vi "FTSMain.vi"() -> ()   [LabVIEW 2020]
uses:
  Popup/Transparent Button.ctl
  Main Menu Selector.ctl
  <instrlib>/PalmSens SDK for LabVIEW 5.10/PalmSens/LiveCurveResult.ctl
  support/PCT FGV CMD.ctl
  support/Message Queue/Message Cluster.ctl
  support/Message Queue/Enqueue Message (Single).vi
  <vilib>/ErrorRing/Error Ring.xnode
  <instrlib>/PalmSens SDK for LabVIEW 5.10/PalmSens/PalmSens.lvclass
  support/Message Queue/Message Queue.lvlib
  Popup/Popup Dialog.lvlib
panel:
  out "Pump Status":bool caption="Pressure"
  out "MFC Status":bool caption="Pressure"
  out "Hiden Status":bool caption="Pressure"
  in  "PS Live Curve Result":T1={"X Label"="Time", "Y Label"="Current", "Name"="Chronoamperometry: CA i vs t", "Index"=0, "Curve Values"={"Values"=array[20001 elements], "Index"=0}}
  in  "Start Motor":bool=TRUE caption="STOP Motor"
  out "Palm Sense Measuring":bool
  out "PS Status":bool caption="Pressure"
  out "User Details":string="Resticted " caption="щн дбегч"
  in  "Multicolumn Listbox":i32(listbox)=1
  out "Motor Status":bool caption="DB"
  in  "Main Menu":T2
  out "String 9":string="V 2.0.2"
  in  "String 7":string="S/N 123456"
  in  "String 6":string="P/N 123456"
  in  "String 5":string="Test Stand"
  out "Time Display":string="12:15:10"
  out "Date Display":string="12.11.2021"
  out "info":string caption="щн дбегч"
  out "Transparent":T3
  in  "Act Log 2":string
  in  "Spare":bool=TRUE caption="StartHeating"
  in  "Test 2":bool=TRUE caption="RUN_Test"
  out "Waveform Graph":dbl[](graph)
  in  "Report":bool
  in  "Timer Run":bool
  in  "CHANNEL 2":bool[](array[boolean])
  out "Display Tab":enum32{"Test", "History"}(tab)
  in  "Start Scan":bool caption="Start Process"
  in  "PS Save Measurements":bool=TRUE caption="RUN_Test"
  out "PS Data":cluster{"X":dbl[], "Y":dbl[]}[](graph)
  out "PS XY Graph":cluster{"X":dbl, "Y":dbl}[](graph)
  out "Waveform Chart 2":dbl[](graph)
  out "SP List Ind":i32(listbox)
  in  "Manual Tab":enum32{"Tango", "PalmSens", "MFC", "Pump"}(tab)
  in  "XYZ Velocity":dbl
  out "Actual Position":cluster{"dX":dbl, "dY":dbl, "dZ":dbl, "dA":dbl}={"dX"=150.0, "dY"=150.0, "dZ"=150.0, "dA"=0.0} caption="Actual Pos\n[mm]"
  in  "Position Mode":string(combo)="Absolute"
  in  "Motor Home":bool=TRUE caption="RUN_Test"
  in  "Set Position":cluster{"dX":dbl, "dY":dbl, "dZ":dbl, "dA":dbl} caption="Set Point\n[mm]" {"dZ" min=-50.0 max=0.0; "dY" min=0.0 max=99.9101; "dX" min=0.0 max=100.586}
  in  "GoToPosition":bool=TRUE caption="RUN_Test"
  in  "PLC Reset":bool caption="RUN_Test"
  in  "PS Scan":bool caption="RUN_Test"
  in  "Start Range":i32(listbox)=6
  in  "Current Range":i32[](listbox)=[3, 4, 5, 6, 7]
  in  "PS Measure Type List":u16(ring) items=["Pretreatment settings (PS)", "Linear Sweep Voltammetry (LSV)", "Differential Pulse Voltammetry (DPV)", "Cyclic Voltammetry (CV)", "Chronoamperometry (CA)", "Chronopotentiometry (CP)", "El Imp Spectroscopy (EIS)"]
  in  "PS Measure Type":T4(tab)
  in  "PS Settings":dbl[](array[numeric])
  in  "LSV Settings":dbl[](array[numeric])
  in  "DPV Settings":dbl[](array[numeric])
  in  "CV Settings":dbl[](array[numeric])
  in  "CA Settings":dbl[](array[numeric])
  in  "CP Settings":dbl[](array[numeric])
  in  "MeasureVsOCP":bool caption="Measure Vs OCP"
  in  "EIS Freq Type":i32(ring) caption="Freq Type" items=["Fixed", "Scan"]
  in  "EIS Scan Type":i32(ring) caption="Scan Type" items=["PGScan", "TimeScan", "Fixed"]
  in  "EIS Settings":dbl[](array[numeric])
  in  "Load PS Config":bool
  in  "SET SP":bool caption="Start Process"
  in  "Selected Gas":string(combo)
  in  "Set Point Options":T5={"Setpoint Value"=0.0, "Mass Flow EU"="", "Setpoint Source"="D", "Valve Mode"="A"}
  in  "Get Info":bool caption="Setting"
  out "Pump Info":T6 {"Direction" items=["CW", "CCW"]; "Speed" format="%03.0f"}
  out "CCW ind":bool
  out "CW ind":bool
  in  "Reverse Direction":bool=TRUE caption="RUN_Test"
  in  "Set CW":bool caption="CW"
  in  "Set CCW":bool caption="CCW"
  in  "Speed":i32 min=0 max=999
  in  "Start Pump":bool=TRUE caption="STOP Motor"
  in  "Row Up":bool caption="Increase"
  in  "Row Down":bool caption="Reduce"
  in  "Set Valves":bool caption="Start Process"
  out "Actual Time":dbl format="%#.1g"
  in  "Valve Time":dbl[](array[numeric])=[10.0, 10.0] min=0.0
  in  "FixActuatorsValve":bool[](array[boolean])=[FALSE, FALSE]
  in  "Manual Pump Select":enum32{"In", "Out"}(radio)
  in  "Stop Process":bool caption="Start Process"
  in  "Start Process":bool
  out "XY Graph":cluster{"X":dbl[], "Y":dbl[]}[](graph)
  out "Test Time 3":dbl caption="Time" format="%<%H:%M:%S>t"
  in  "Test Step Done":i32(listbox)=15
  out "Act Log":string
  in  "Test Types":string(tree)
  out "DAQ timeout":bool
  out "DAQ Status":bool caption="PLC"
  out "PLC Heartbeat":bool
  in  "Reset Error":bool
  out "on Test":bool caption="Pressure"
  out "DB":bool=TRUE caption="Pressure"
  out "PLC":bool caption="Pressure"
  out "Alarm Display":string="Operator: Eugene, \nLocation: Chemistry Lab" caption="щн дбегч"
  out "Timer":cluster{dbl, dbl, dbl}(knob)={4.800000000000001, 9.686666666666666, 5.2} scale=0.0..11.0 scale format="%#_1g"
  out "Test Time 2":dbl=3665400506.523932 caption="Time" format="%<%H:%M:%S>T"
  out "status":string="automatic test" caption="щн дбегч"
  in  "Swich V Tab":bool
  out "LOG":string="automatic test" caption="щн дбегч"
  in  "Switch Main Tab":enum32{"Test", "History"}(radio) caption="Procedures"
  in  "Sign In":bool
  in  "Test Setting":bool caption="Setting"
  in  "HW Configuration":bool
  in  "Exit":bool
  in  "Start":bool caption="RUN_Test"
  # "90"
  # "180"
  # "TIME"
  # "STATUS"
  # "TEST"
  # "HISTORY"
  # "SAVE"
  # "UPDATE"
  # "RESULTS"
  # "GAGES"
  # "FRONT"
  # "BACK"
  # "RPM"
  # "MANUAL CONTROL"
  # "Hiden Scan"
  # "Go to Position"
  # "RESET"
  # "HOME"
  # "ConditioningPotential"
  # "ConditioningTime"
  # "DepositionPotential"
  # "DepositionTime"
  # "EquilibrationTime"
  # "BeginPotential"
  # "EndPotential"
  # "StepPotential"
  # "Scanrate"
  # "BeginPotential"
  # "EndPotential"
  # "StepPotential"
  # "Scanrate"
  # "PulsePotential"
  # "PulseTime"
  # "BeginPotential"
  # "Vtx1Potential"
  # "Vtx2Potential"
  # "StepPotential"
  # "Scanrate"
  # "nScans"
  # "Potential"
  # "IntervalTime"
  # "RunTime"
  # "Current"
  # "AppliedCurrentRange"
  # "RunTime"
  # "IntervalTime"
  # "EquilibrationTime"
  # "Eac"
  # "BeginPotential"
  # "EndPotential"
  # "StepPotential"
  # "Potential"
  # "MaxFrequency"
  # "MinFrequency"
  # "nFrequencies"
  # "SamplingTime"
  # "MaxEqTime"
  # "RunTime"
  # "Interval Time"
  # "Stability Criterion"
  # "OCP Max Time"
  # "Direction"
  # "CW"
  # "CCW"
  # "Speed"
  # "Increase"
  # "Reduce"
  # "1 RPM"
  # "1 RPM"
  # "Get Info"
  # "VALVE"
  # "Time [s]"
  # "In"
  # "Out"
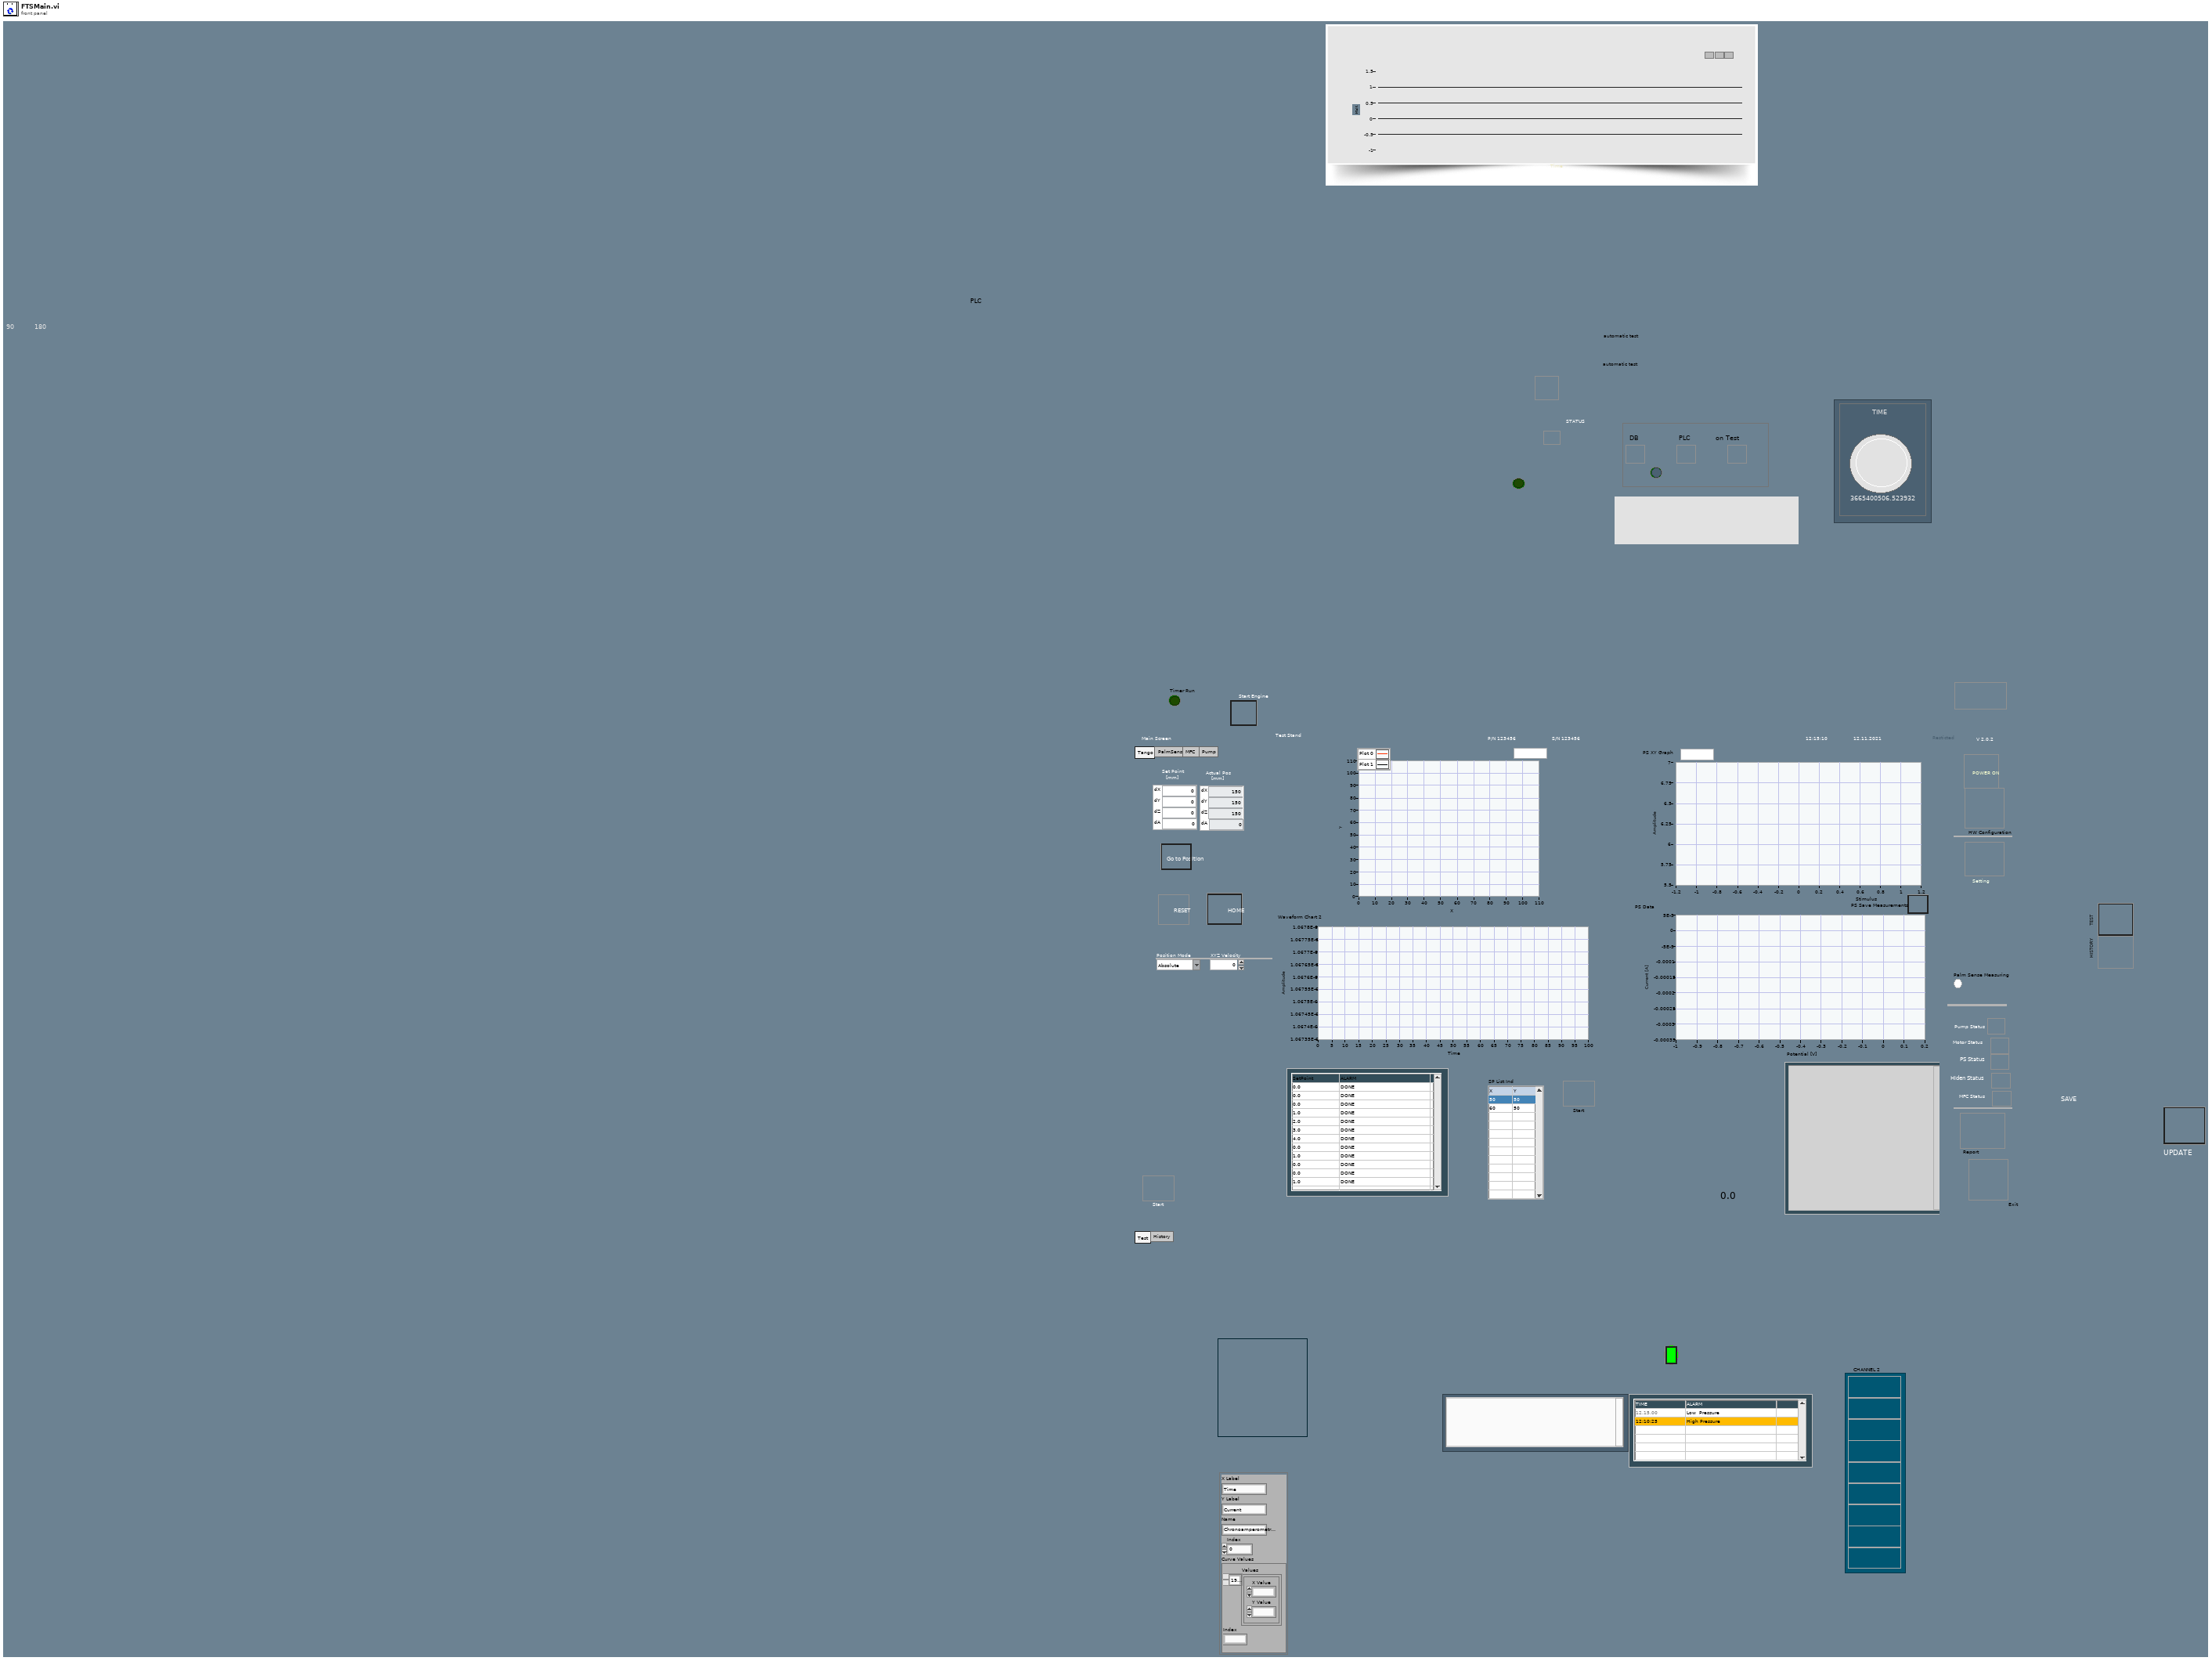
[diagram p1: front panel]
types:
  T1 = typedef "LiveCurveResult.ctl" = cluster{"X Label":string, "Y Label":string, "Name":string, "Index":i16, "Curve Values":cluster{"Values":cluster{"X Value":dbl, "Y Value":dbl}[], "Index":i16}}
  T2 = typedef "Main Menu Selector.ctl" = enum16{"Main Screen", "Test Setting", "Calibration", "History", "Admin", "Switch User", "About", "Exit"}
  T3 = typedef "Popup Dialog.lvlib/Transparent Button.ctl" = bool
  T4 = enum32{"Pretreatment settings (PS)", "Linear Sweep Voltammetry (LSV)", "Differential Pulse Voltammetry (DPV)", "Cyclic Voltammetry (CV)", "Chronoamperometry (CA)", "Chronopotentiometry (CP)", "El Imp Spectroscopy (EIS)"}
  T5 = cluster{"Setpoint Value":dbl, "Mass Flow EU":string, "Setpoint Source":string, "Valve Mode":string}
  T6 = cluster{"Pump Type":string, "Speed":i32, "Direction":u16, "Running":bool}
  T7 = typedef "PCT Data REFs.ctl" = cluster{"PLC AI Notifier":refnum<notifier>, "PS Data Queue":refnum<queue>, "BTN Queue":refnum<queue>, "PLC DI notifier":refnum<notifier>, "Timer notifier":refnum<notifier>, "DMM PS":refnum<notifier>, "DMM Gages":refnum<notifier>, "XYZ notifier":refnum<notifier>, "Test Notifier":refnum<notifier>, "Scanner notifier":refnum<notifier>, "OPC Notifier":refnum<notifier>, "HIDEN queue":refnum<queue>}
  T8 = typedef "Message Queue.lvlib/All Message Queues.ctl" = cluster{"UI":refnum<queue>, "Logging":refnum<queue>, "LOG":refnum<queue>, "ALARM":refnum<queue>, "Test":refnum<queue>, "Answer":refnum<queue>, "PLC":refnum<queue>, "DB":refnum<queue>, "Report":refnum<queue>, "OPC":refnum<queue>, "Procedure":refnum<queue>, "PalmSens":refnum<queue>, "SYS 7000 Reader":refnum<queue>, "SWITCH":refnum<queue>, "MOTOR":refnum<queue>, "MOTION":refnum<queue>, "HIDEN":refnum<queue>, "VALVE":refnum<queue>, "MFC":refnum<queue>, "PUMP IN":refnum<queue>, "PUMP OUT":refnum<queue>}
  T9 = typedef "PCT FGV CMD.ctl" = enum16{"INIT", "GET", "SET"}
  T10 = cluster{"Writer Queue":refnum<queue>, "Timeout":dbl[], "Status":bool[]}
  T11 = typedef "LVPoint32TypeDef.ctl" = cluster{"Horizontal":i32, "Vertical":i32}
  T12 = typedef "LVRowAndColumnTypeDef.ctl" = cluster{"Row":i32, "Column":i32}
  T13 = typedef "MeasurementResults.ctl" = T1[]
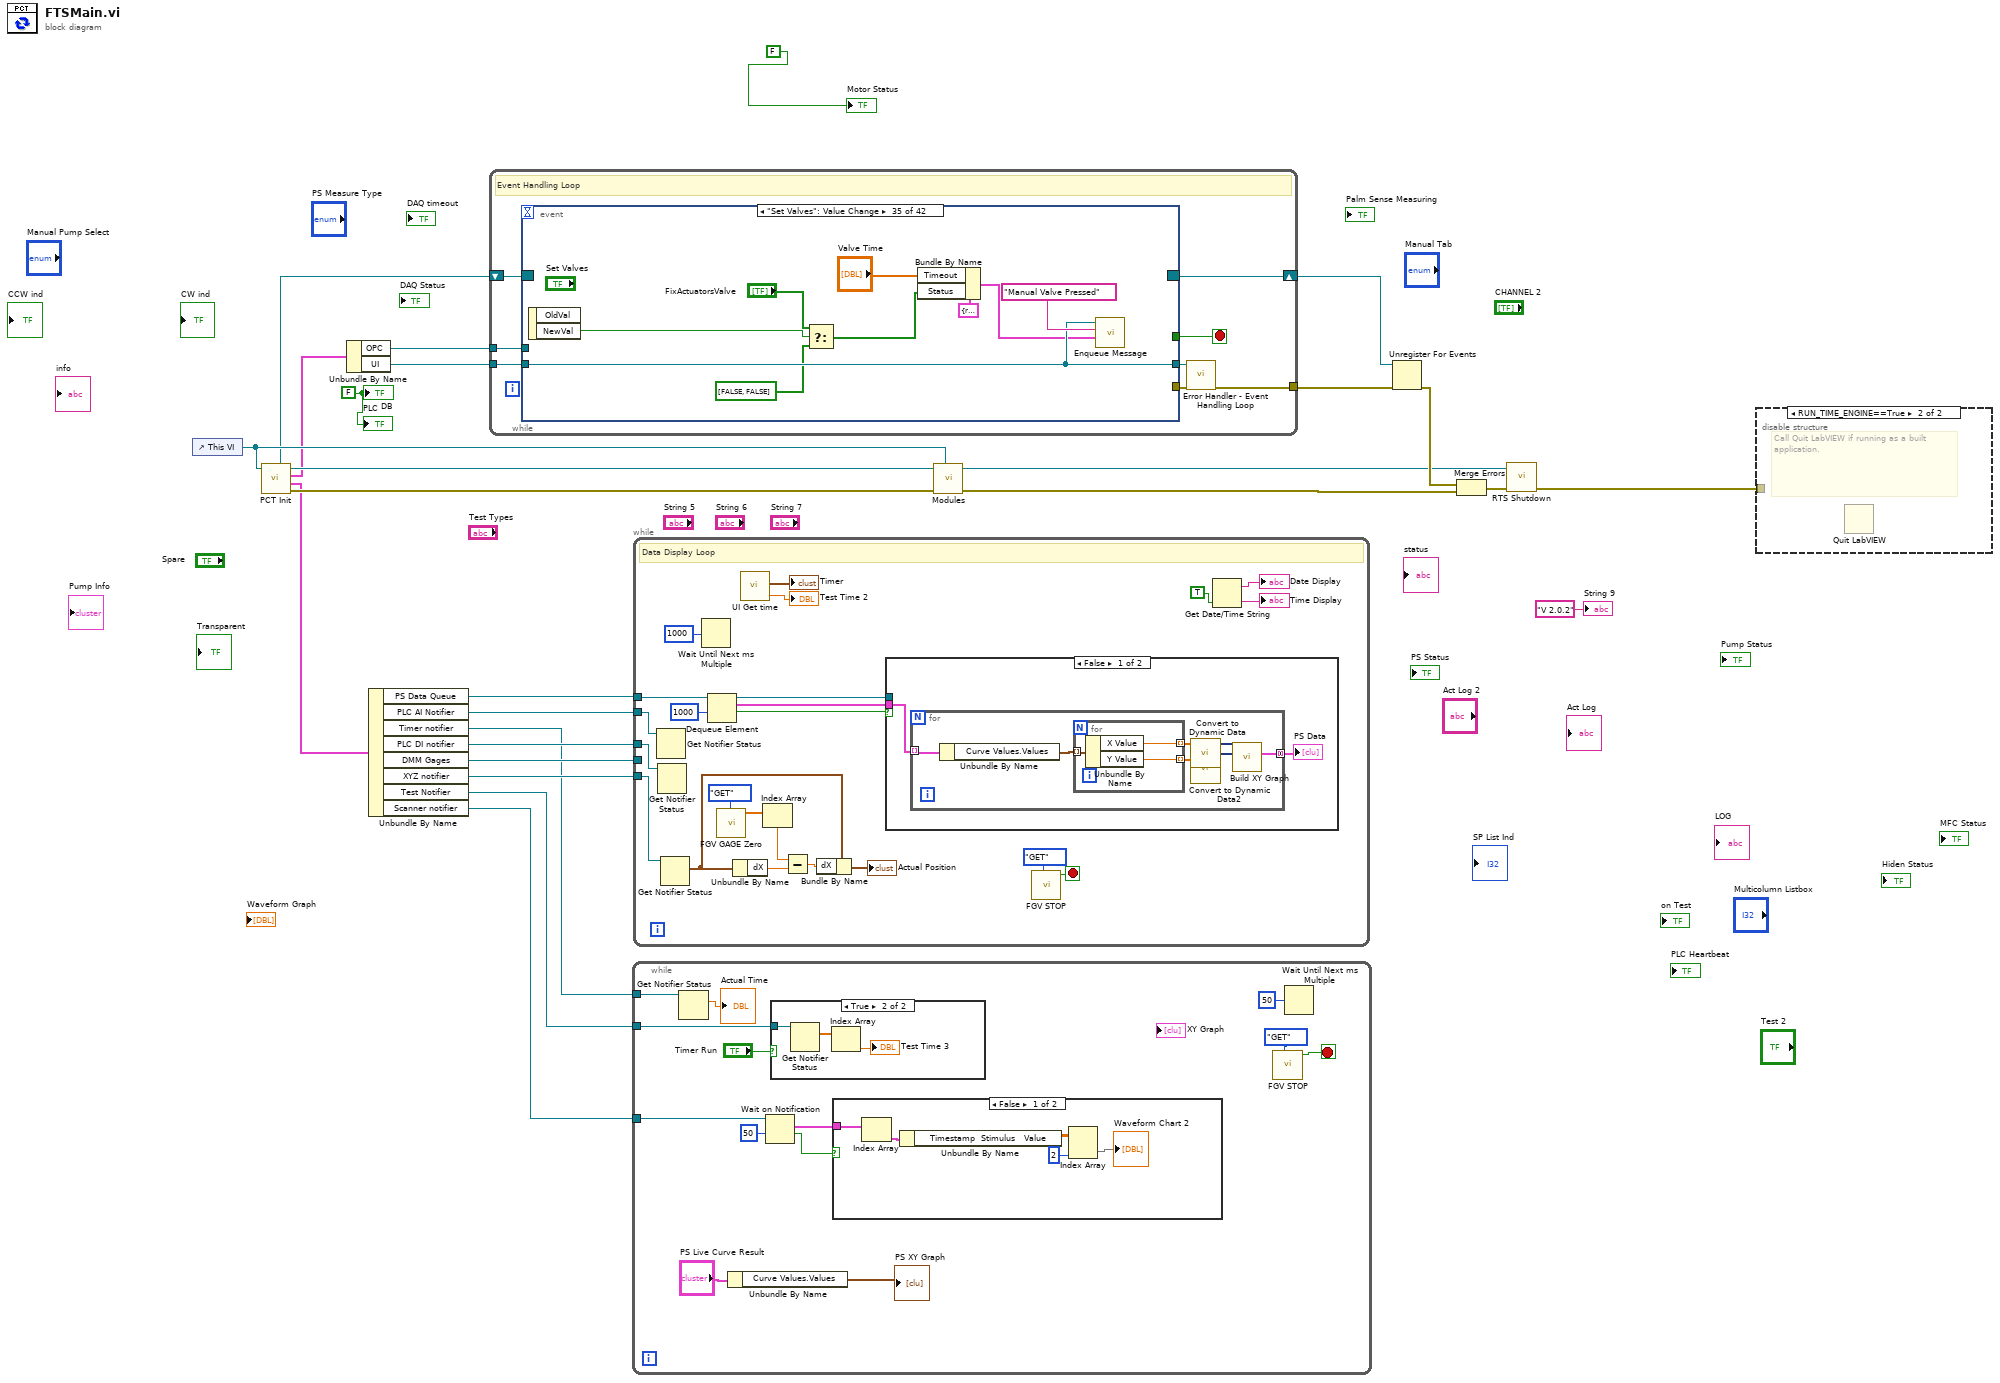
[diagram p0: block diagram]
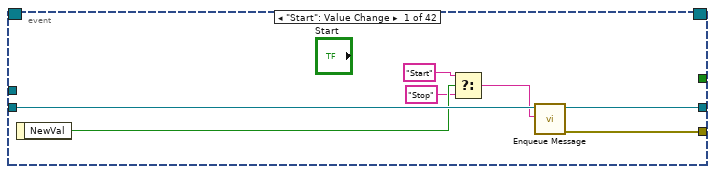
[diagram p6: hidden frame]
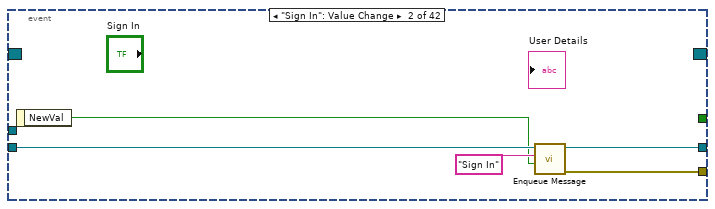
[diagram p7: hidden frame]
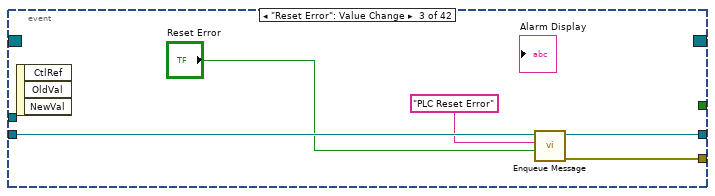
[diagram p8: hidden frame]
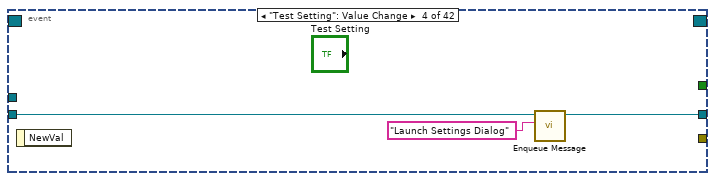
[diagram p9: hidden frame]
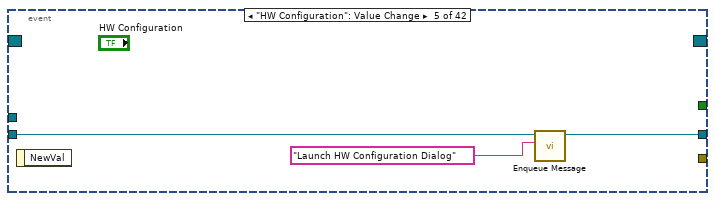
[diagram p10: hidden frame]
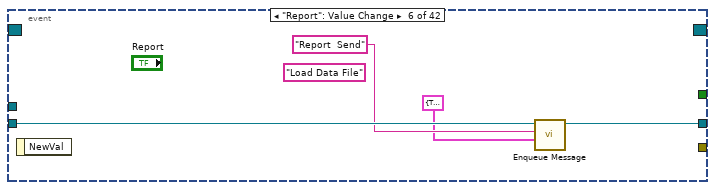
[diagram p11: hidden frame]
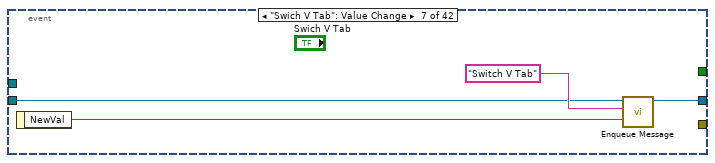
[diagram p12: hidden frame]
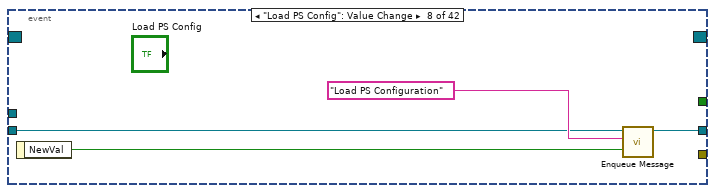
[diagram p13: hidden frame]
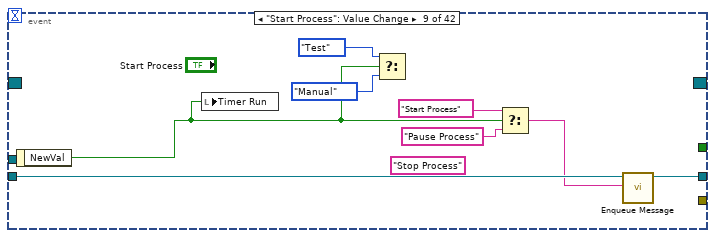
[diagram p14: hidden frame]
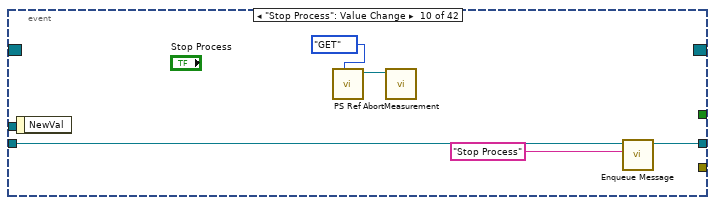
[diagram p15: hidden frame]
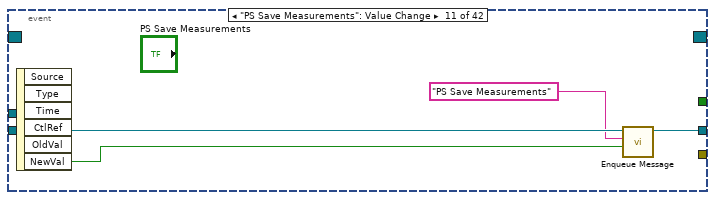
[diagram p16: hidden frame]
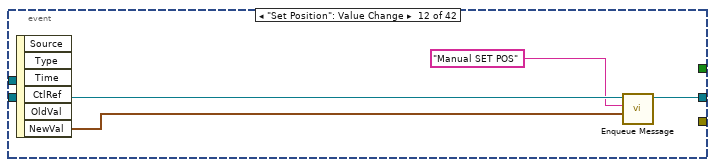
[diagram p17: hidden frame]
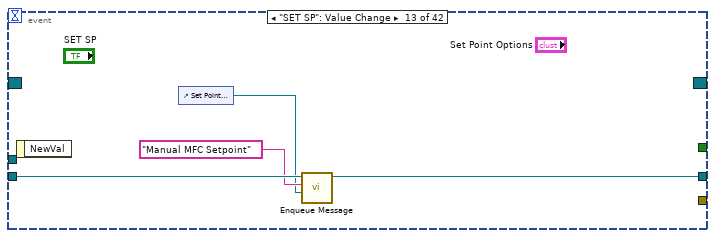
[diagram p18: hidden frame]
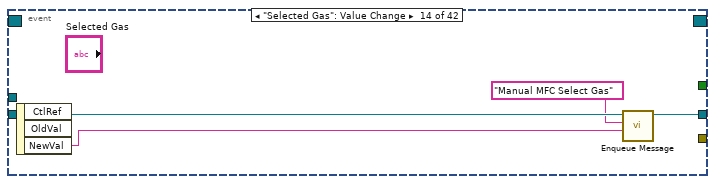
[diagram p19: hidden frame]
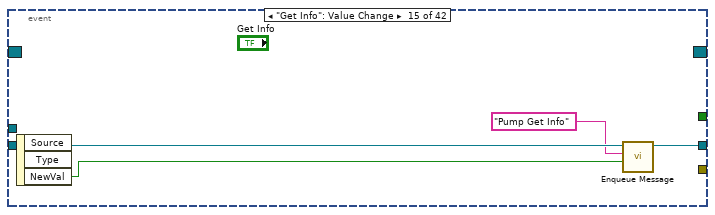
[diagram p20: hidden frame]
diagram:
  w10 = FALSE ("DB")
  n1 = control-ref of="This VI"() -> (w16:refnum<vi>)
  n2 = call "PCT Init.vi"("VI in"=w16) -> ("error out"=w21:errorcluster, "Data REF"=w18:T7, "Message Queues out"=w13:T8, "User Event out"=w20:refnum<user-event>, "Event Registration Refnum"=w12:refnum<event-registration>)  [unwired: 6 in]
  n3 = Unbundle By Name(w13) -> ("OPC"=w3:refnum<queue>, "UI"=w17:refnum<queue>)
  n4 = Unbundle By Name(w18) -> ("PS Data Queue"=w14:refnum<queue>, "PLC AI Notifier"=w11:refnum<notifier>, "Timer notifier"=w1:refnum<notifier>, "PLC DI notifier"=w6:refnum<notifier>, "DMM Gages"=w5:refnum<notifier>, "XYZ notifier"=w8:refnum<notifier>, "Test Notifier"=w9:refnum<notifier>, "Scanner notifier"=w2:refnum<notifier>)
  n5 = while {
    tunnel: w17 -> [w33]
    tunnel: [w30] -> w26
    shift-right: [w32] -> w25
    shift-left: w12 -> [w34]
    tunnel: w3 -> [w27]
    stop <- w31 stop-if-true
    # "Event Handling Loop"
    n6 = event shown="[34] \"Set Valves\": Value Change" {
      selector: w34 -> [_ _ _ _ _ _ _ _ _ _ _ _ _ _ _ _ _ _ _ _ _ _ _ _ _ _ _ _ _ _ _ _ _ _ _ _ _ _ _ _ _ _]
      dyn-events: [_ _ _ _ _ _ _ _ _ _ _ _ _ _ _ _ _ _ _ _ _ _ _ _ _ _ _ _ _ _ _ _ _ _ _ _ _ _ _ _ _ _] -> w32
      timeout: _ -> [_ _ _ _ _ _ _ _ _ _ _ _ _ _ _ _ _ _ _ _ _ _ _ _ _ _ _ _ _ _ _ _ _ _ _ _ _ _ _ _ _ _]
      tunnel: [_ _ _ _ _ _ _ _ _ _ _ _ _ _ _ _ _ _ _ _ _ _ _ _ _ _ _ _ _ _ _ _ TRUE ("Discard?") _ _ _ _ _ _ _ _ _] -> w31
      tunnel: w33 -> [w41 w46 w51 w53 w56 w61 w64 w68 w77 w82 w86 w90 w94 w98 w102 w106 w109 w114 w119 w123 w135 w143 w150 w160 w168 w172 w182 w186 w190 w194 w197 w201 w205 w210 w218 w222 w226 w236 w253 w257 w264 w272]
      tunnel: [w40 w45 w50 _ _ _ _ _ _ _ _ _ _ _ _ _ _ _ _ _ _ _ _ _ _ _ _ _ _ w192 _ w203 _ _ _ _ _ _ _ _ _ _] -> w29
      tunnel: [w39 w44 w49 w52 w55 w60 w63 w67 w76 w81 w85 w89 w93 w97 w101 w105 w108 w113 w118 w122 w134 w142 w149 w159 w166 w171 w181 w185 w189 w193 w197 w200 w205 w210 w218 w222 w223 w235 w252 w256 w264 w272] -> w28
      tunnel: w27 -> [_ _ _ _ _ _ _ _ _ _ _ _ _ _ _ _ _ _ _ _ _ _ w146 _ _ _ _ _ _ _ _ _ _ _ _ _ _ _ _ _ _ _]
      event "Start": Value Change {
        n7 = event-data() -> ("NewVal"=w38:bool)  [unwired: 1 in]
        n8 = Select(t="Start" ("Message"), s=w38, f="Stop") -> (s? t:f=w35:string)
        n9 = call-poly "Enqueue Message.vi"("Message"=w35, "Message Queue"=w41) -> ("error out"=w40:errorcluster, "dup Message Queue"=w39:refnum<queue>)  [unwired: 8 in]
      }
      event "Sign In": Value Change {
        n10 = event-data() -> ("NewVal"=w42:bool)  [unwired: 1 in]
        n11 = call-poly "Enqueue Message.vi"("Message Data"=w42, "Message"="Sign In", "Message Queue"=w46) -> ("error out"=w45:errorcluster, "dup Message Queue"=w44:refnum<queue>)  [unwired: 7 in]
      }
      event "Reset Error": Value Change {
        n12 = event-data() -> ()  [unwired: 1 in, 3 out]
        n13 = call-poly "Enqueue Message.vi"("Message Data"="Reset Error", "Message"="PLC Reset Error", "Message Queue"=w51) -> ("error out"=w50:errorcluster, "dup Message Queue"=w49:refnum<queue>)  [unwired: 7 in]
      }
      event "Test Setting": Value Change {
        n14 = event-data() -> ()  [unwired: 1 in, 1 out]
        n15 = call-poly "Enqueue Message.vi"("Message"="Launch Settings Dialog", "Message Queue"=w53) -> ("dup Message Queue"=w52:refnum<queue>)  [unwired: 8 in, 1 out]
      }
      event "HW Configuration": Value Change {
        n16 = event-data() -> ()  [unwired: 1 in, 1 out]
        n17 = call-poly "Enqueue Message.vi"("Message"="Launch HW Configuration Dialog", "Message Queue"=w56) -> ("dup Message Queue"=w55:refnum<queue>)  [unwired: 8 in, 1 out]
      }
      event "Report": Value Change {
        (unwired) "Load Data File" ("Message")
        n18 = event-data() -> ()  [unwired: 1 in, 1 out]
        n19 = call-poly "Enqueue Message.vi"("Message Data"=cluster{bool, "Data File Path":path} {TRUE, "Data File Path"=path ""}, "Message"="Report  Send", "Message Queue"=w61) -> ("dup Message Queue"=w60:refnum<queue>)  [unwired: 7 in, 1 out]
      }
      event "Swich V Tab": Value Change {
        n20 = event-data() -> ("NewVal"=w62:bool)  [unwired: 1 in]
        n21 = call-poly "Enqueue Message.vi"("Message Data"=w62, "Message"="Switch V Tab", "Message Queue"=w64) -> ("dup Message Queue"=w63:refnum<queue>)  [unwired: 7 in, 1 out]
      }
      event "Load PS Config": Value Change {
        n22 = event-data() -> ("NewVal"=w66:bool)  [unwired: 1 in]
        n23 = call-poly "Enqueue Message.vi"("Message Data"=w66, "Message"="Load PS Configuration", "Message Queue"=w68) -> ("dup Message Queue"=w67:refnum<queue>)  [unwired: 7 in, 1 out]
      }
      event "Start Process": Value Change {
        (unwired) "Stop Process" ("Message")
        n24 = event-data() -> ("NewVal"=w72:bool)  [unwired: 1 in]
        n25 = local write "Timer Run"(w72) -> ()
        n26 = Select(t=enum32{"Manual", "Test"}."Test" ("Manual Tab"), s=w72, f=enum32{"Manual", "Test"}."Manual" ("Manual Tab")) -> ()  [unwired: 1 out]
        n27 = Select(t="Start Process" ("Message"), s=w72, f="Pause Process" ("Message")) -> (s? t:f=w74:string)
        n28 = call-poly "Enqueue Message.vi"("Message"=w74, "Message Queue"=w77) -> ("dup Message Queue"=w76:refnum<queue>)  [unwired: 8 in, 1 out]
      }
      event "Stop Process": Value Change {
        n29 = event-data() -> ()  [unwired: 1 in, 1 out]
        n30 = call "PS Ref.vi"("CMD"=PCT_FGV_CMD."GET") -> ("PalmSens.lvclass out"=w79:refnum<class "PalmSens.lvclass">)  [unwired: 9 in, 1 out]
        n31 = call-dynamic "AbortMeasurement.vi"("PalmSens in"=w79) -> ()  [unwired: 9 in, 2 out]
        n32 = call-poly "Enqueue Message.vi"("Message"="Stop Process", "Message Queue"=w82) -> ("dup Message Queue"=w81:refnum<queue>)  [unwired: 8 in, 1 out]
      }
      event "PS Save Measurements": Value Change {
        n33 = event-data() -> ("NewVal"=w83:bool)  [unwired: 1 in, 5 out]
        n34 = call-poly "Enqueue Message.vi"("Message Data"=w83, "Message"="PS Save Measurements", "Message Queue"=w86) -> ("dup Message Queue"=w85:refnum<queue>)  [unwired: 7 in, 1 out]
      }
      event "Set Position": Value Change {
        n35 = event-data() -> ("NewVal"=w87:cluster{"dX":dbl, "dY":dbl, "dZ":dbl, "dA":dbl})  [unwired: 1 in, 5 out]
        n36 = call-poly "Enqueue Message.vi"("Message Data"=w87, "Message"="Manual SET POS", "Message Queue"=w90) -> ("dup Message Queue"=w89:refnum<queue>)  [unwired: 7 in, 1 out]
      }
      event "SET SP": Value Change {
        n37 = event-data() -> ()  [unwired: 1 in, 1 out]
        n38 = control-ref of="Set Point Options"() -> (w91:refnum<vi>)
        n39 = call-poly "Enqueue Message.vi"("Message Data"=w91, "Message"="Manual MFC Setpoint", "Message Queue"=w94) -> ("dup Message Queue"=w93:refnum<queue>)  [unwired: 7 in, 1 out]
      }
      event "Selected Gas": Value Change {
        n40 = event-data() -> ("NewVal"=w95:string)  [unwired: 1 in, 2 out]
        n41 = call-poly "Enqueue Message.vi"("Message Data"=w95, "Message"="Manual MFC Select Gas", "Message Queue"=w98) -> ("dup Message Queue"=w97:refnum<queue>)  [unwired: 7 in, 1 out]
      }
      event "Get Info": Value Change {
        n42 = event-data() -> ("NewVal"=w99:bool)  [unwired: 1 in, 2 out]
        n43 = call-poly "Enqueue Message.vi"("Message Data"=w99, "Message"="Pump Get Info", "Message Queue"=w102) -> ("dup Message Queue"=w101:refnum<queue>)  [unwired: 7 in, 1 out]
      }
      event "Speed": Value Change {
        n44 = event-data() -> ("NewVal"=w103:i32)  [unwired: 1 in, 2 out]
        n45 = call-poly "Enqueue Message.vi"("Message Data"=w103, "Message"="Pump Set Speed", "Message Queue"=w106) -> ("dup Message Queue"=w105:refnum<queue>)  [unwired: 7 in, 1 out]
      }
      event "Reverse Direction": Value Change {
        n46 = event-data() -> ()  [unwired: 1 in, 3 out]
        n47 = call-poly "Enqueue Message.vi"("Message"="Pump Reverse Direction", "Message Queue"=w109) -> ("dup Message Queue"=w108:refnum<queue>)  [unwired: 8 in, 1 out]
      }
      event "Row Up", "Row Down": Value Change {
        n48 = event-data() -> ("CtlRef"=w111:refnum<vi>)  [unwired: 1 in, 2 out]
        n49 = property class="Bool (strict)"(reference=w111) -> ("Caption.Text"=w110:string)  [unwired: 1 in, 2 out]
        n50 = call-poly "Enqueue Message.vi"("Message Data"=w110, "Message"="Pump Change Speed", "Message Queue"=w114) -> ("dup Message Queue"=w113:refnum<queue>)  [unwired: 7 in, 1 out]
      }
      event "Set CCW", "Set CW": Value Change {
        n51 = event-data() -> ("CtlRef"=w116:refnum<vi>)  [unwired: 1 in, 2 out]
        n52 = property class="Bool"(reference=w116) -> ("Caption.Text"=w115:string)  [unwired: 1 in, 2 out]
        n53 = call-poly "Enqueue Message.vi"("Message Data"=w115, "Message"="Pump Set Direction", "Message Queue"=w119) -> ("dup Message Queue"=w118:refnum<queue>)  [unwired: 7 in, 1 out]
      }
      event "Start Pump": Value Change {
        n54 = event-data() -> ("NewVal"=w120:bool)  [unwired: 1 in]
        n55 = call-poly "Enqueue Message.vi"("Message Data"=w120, "Message"="Pump Start", "Message Queue"=w123) -> ("dup Message Queue"=w122:refnum<queue>)  [unwired: 7 in, 1 out]
      }
      event "Test Types": Double Click {
        (unwired) "DB Get Tests" ("Message")
        # "\"Load Data File\""
        n56 = event-data() -> ("CtlRef"=w130:refnum<vi>, "Tag"=w129:string)  [unwired: 1 in]
        n57 = invoke class="Tree (strict)" method="Navigate Tree.Get Parent"(reference=w130, "tag"=w129) -> ()  [unwired: 2 in, 4 out]
        n58 = property on="Property Node" class="Tree (strict)" props=["Active Item Tag", "Active Item Row Number", "ActiveColNum", "Cell String", "ActiveColNum", "Cell String", "ActiveColNum", "Cell String"](reference=w130, "Active Item Tag"=w129, "ActiveColNum"=7 ("Active Cell:Active Column Number"), "ActiveColNum"=9 ("Active Cell:Active Column Number"), "ActiveColNum"=2 ("Active Cell:Active Column Number")) -> ("Cell String"=w128:string, "Cell String"=w125:string, "Cell String"=w124:string)  [unwired: 1 in, 3 out]
        n59 = String To Path(string=w128) -> (path=w127:path)
        n60 = Build Array(w125, w124) -> ()  [unwired: 1 out]
        n61 = Empty String/Path?(string/path=w127) -> (empty?=w126:bool)
        n62 = case shown="False" w126 {
          tunnel: w135 -> [w138 w139]
          tunnel: [w137 w139] -> w134
          frame False {
            n63 = call-poly "Enqueue Message.vi"("Message"="Load RES File", "Message Queue"=w138) -> ("dup Message Queue"=w137:refnum<queue>)  [unwired: 8 in, 1 out]
          }
          frame True {
          }
        }
      }
      event "PLC Reset": Value Change {
        n64 = event-data() -> ("NewVal"=w140:bool)  [unwired: 1 in]
        n65 = call-poly "Enqueue Message.vi"("Message Data"=w140, "Message"="Manual SET Reset", "Message Queue"=w143) -> ("dup Message Queue"=w142:refnum<queue>)  [unwired: 7 in, 1 out]
      }
      event "Start Motor": Value Change {
        n66 = event-data() -> ("NewVal"=w147:bool)  [unwired: 1 in]
        n67 = call-poly "Enqueue Message.vi"("Priority Message? (F)"=TRUE, "Message"="Send Response", "Message Queue"=w146) -> ()  [unwired: 7 in, 2 out]
        n68 = call-poly "Enqueue Message.vi"("Message Data"=w147, "Message"="Manual Motor Stop", "Message Queue"=w150) -> ("dup Message Queue"=w149:refnum<queue>)  [unwired: 7 in, 1 out]
      }
      event "Test Step Done": Mouse Down {
        n69 = event-data() -> ("Mods.Double Click"=w158:bool, "CtlRef"=w157:refnum<vi>, "Coords"=w153:T11)  [unwired: 1 in]
        n70 = property class="MCListbox (strict)"(reference=w157) -> ("ItemNames"=w156:string[][])  [unwired: 1 in, 2 out]
        n71 = invoke class="MCListbox (strict)" method="Point To Row Column"(reference=w157, "Point"=w153) -> ("CellPosition"=w152:T12)  [unwired: 5 in, 6 out]
        n72 = Unbundle By Name(w152) -> ("Row"=w151:i32)
        n73 = Index Array(array=w156, index (row)=w151, index (col)=0 ("disabled index (col)")) -> (element=w155:string)
        n74 = case shown="True" w158 {
          tunnel: w160 -> [w161 w165]
          tunnel: [w161 w164] -> w159
          tunnel: w155 -> [_ w162]
          frame False {
          }
          frame True {
            n75 = call-poly "Enqueue Message.vi"("Message Data"=w162, "Message"="Load Data File", "Message Queue"=w165) -> ("dup Message Queue"=w164:refnum<queue>)  [unwired: 7 in, 1 out]
          }
        }
      }
      event "Motor Home": Value Change {
        n76 = event-data() -> ()  [unwired: 1 in, 1 out]
        n77 = call-poly "Enqueue Message.vi"("Message Data"=FALSE, "Message"="Send PLC Home", "Message Queue"=w168) -> ("dup Message Queue"=w166:refnum<queue>)  [unwired: 7 in, 1 out]
      }
      event "PS Scan": Value Change {
        n78 = event-data() -> ("NewVal"=w170:bool)  [unwired: 1 in]
        n79 = case shown="True" w170 {
          tunnel: w172 -> [w173 w178]
          tunnel: [w173 w177] -> w171
          frame False {
            n80 = call "PS Ref.vi"("CMD"=PCT_FGV_CMD."GET") -> ("PalmSens.lvclass out"=w175:refnum<class "PalmSens.lvclass">)  [unwired: 9 in, 1 out]
            n81 = call-dynamic "AbortMeasurement.vi"("PalmSens in"=w175) -> ()  [unwired: 9 in, 2 out]
          }
          frame True {
            n82 = call-poly "Enqueue Message.vi"("Message"="Manual PS Scan", "Message Queue"=w178) -> ("dup Message Queue"=w177:refnum<queue>)  [unwired: 8 in, 1 out]
          }
        }
      }
      event "Start Scan": Value Change {
        n83 = event-data() -> ()  [unwired: 1 in, 1 out]
        n84 = call-poly "Enqueue Message.vi"("Message Data"="Start Scan", "Message"="Manual Start Scan", "Message Queue"=w182) -> ("dup Message Queue"=w181:refnum<queue>)  [unwired: 7 in, 1 out]
      }
      event "Position Mode": Value Change {
        n85 = event-data() -> ()  [unwired: 1 in, 1 out]
        n86 = call-poly "Enqueue Message.vi"("Message Data"="Position Mode", "Message"="Position Mode", "Message Queue"=w186) -> ("dup Message Queue"=w185:refnum<queue>)  [unwired: 7 in, 1 out]
      }
      event "GoToPosition": Value Change {
        # "each 1 increment in pos is 50 microns vertical movement of the beam"
        n87 = event-data() -> ()  [unwired: 1 in, 1 out]
        n88 = call-poly "Enqueue Message.vi"("Message Data"="Set Position", "Message"="Manual GO POS", "Message Queue"=w190) -> ("dup Message Queue"=w189:refnum<queue>)  [unwired: 7 in, 1 out]
      }
      event Panel Close? {
        n89 = event-data() -> ()  [unwired: 1 in, 1 out]
        n90 = call-poly "Enqueue Message.vi"("Priority Message? (F)"=TRUE, "Message"="Confirm Quit", "Message Queue"=w194) -> ("error out"=w192:errorcluster, "dup Message Queue"=w193:refnum<queue>)  [unwired: 7 in]
        n91 = event-data("Discard?"=TRUE) -> ()  [unwired: 1 in, 1 out]
      }
      event Application Instance Close {
        n92 = event-data() -> ()  [unwired: 1 in, 1 out]
      }
      event "Exit": Value Change {
        w199 = TRUE  # Priority Message
        n93 = event-data() -> ()  [unwired: 1 in, 1 out]
        n94 = xnode "Error Ring"() -> ("error out"=w198:errorcluster)
        n95 = call-poly "Enqueue Message.vi"("Priority Message? (F)"=w199, "Message Data"=w198, "Message"="Exit", "Message Queue"=w201) -> ("error out"=w203:errorcluster, "dup Message Queue"=w200:refnum<queue>)  [unwired: 6 in]
      }
      event User Event {
        n96 = event-data() -> ()  [unwired: 1 in, 1 out]
        n97 = local write "status"("Exit" ("Exit String")) -> ()
      }
      event "Switch Main Tab": Value Change {
        (unwired) refnum<vi> refnum ("Display Tab")
        (unwired) enum32{"Test", "History"}."Test" ("Switch Main Tab")
        n98 = event-data() -> ()  [unwired: 1 in, 1 out]
        n99 = call-poly "Enqueue Message.vi"("Message Data"="Switch Main Tab", "Message"="Main Tab Switch", "Message Queue"=w210) -> ()  [unwired: 7 in, 2 out]
        "Display Tab" <- "Switch Main Tab"
      }
      event "Set Valves": Value Change {
        n100 = event-data() -> ("NewVal"=w214:bool)  [unwired: 1 in, 1 out]
        n101 = Select(t="FixActuatorsValve", s=w214, f=bool[] [FALSE, FALSE] ("FixActuatorsValve")) -> (s? t:f=w211:bool[])
        n102 = Bundle By Name(cluster=T10 {"Writer Queue"=refnum, "Timeout"=[], "Status"=[]}, "Timeout"="Valve Time", "Status"=w211) -> (w216:T10)
        n103 = call-poly "Enqueue Message.vi"("Message Data"=w216, "Message"="Manual Valve Pressed", "Message Queue"=w218) -> ()  [unwired: 7 in, 2 out]
      }
      event Value Change {
        (unwired) Main_Menu_Selector."Main Screen" ("Main Menu")
        n104 = event-data() -> ("NewVal"=w220:T2)  [unwired: 1 in]
        n105 = call-poly "Enqueue Message.vi"("Message Data"=w220, "Message"="Main Menu Value Change", "Message Queue"=w222) -> ()  [unwired: 7 in, 2 out]
      }
      event "PS Measure Type List": Value Change {
        n106 = event-data() -> ("CtlRef"=w225:refnum<vi>)  [unwired: 1 in]
        n107 = property class="Ring (strict)"(reference=w225) -> ("RingText.Text"=w224:string)  [unwired: 1 in, 2 out]
        n108 = call-poly "Enqueue Message.vi"("Message Data"=w224, "Message"="PS Measure Type Update", "Message Queue"=w226) -> ("dup Message Queue"=w223:refnum<queue>)  [unwired: 7 in, 1 out]
      }
      event "EIS Settings", "CP Settings", "CA Settings", "CV Settings", "DPV Settings", "LSV Settings", "PS Settings": Value Change {
        n109 = event-data() -> ("NewVal"=w229:dbl[])  [unwired: 1 in, 2 out]
        n110 = property on="PS Measure Type List" class="Ring (strict)"() -> ("RingText.Text"=w230:string)  [unwired: 2 in, 2 out]
        n111 = call "PS long Name to Short.vi"("String"=w230) -> ("whole match"=w231:string)  [unwired: 10 in]
        n112 = Format Into String(format string="%s Scan", w231) -> (resulting string=w234:string)  [unwired: 2 in, 1 out]
        n113 = call "FGV Parameters.vi"("CMD"=PCT_FGV_CMD."SET", "input"=w229, "Key"=w234) -> ("error out"=w228:errorcluster)  [unwired: 6 in, 2 out]
        n114 = call-poly "Enqueue Message.vi"("error in (no error)"=w228, "Message"="PS Scan Update", "Message Queue"=w236) -> ("dup Message Queue"=w235:refnum<queue>)  [unwired: 7 in, 1 out]
      }
      event "EIS Scan Type", "EIS Freq Type", "MeasureVsOCP": Value Change {
        n115 = event-data() -> ()  [unwired: 1 in, 6 out]
        n116 = property on="PS Measure Type List" class="Ring (strict)"() -> ("RingText.Text"=w247:string)  [unwired: 2 in, 2 out]
        n117 = call "PS long Name to Short.vi"("String"=w247) -> ("whole match"=w248:string)  [unwired: 10 in]
        n118 = Boolean To (0,1)(Boolean="MeasureVsOCP") -> (0, 1=w242:i16)
        n119 = Build Array("EIS Scan Type", "EIS Freq Type", w242) -> (w239:i32[])
        n120 = Format Into String(format string="%s Scan", w248) -> (resulting string=w251:string)  [unwired: 2 in, 1 out]
        n121 = Replace Array Subset(array="EIS Settings", new element=w239, index=15) -> (w238:dbl[])
        n122 = call "FGV Parameters.vi"("CMD"=PCT_FGV_CMD."SET", "input"=w238, "Key"=w251) -> ("error out"=w246:errorcluster)  [unwired: 6 in, 2 out]
        n123 = call-poly "Enqueue Message.vi"("error in (no error)"=w246, "Message"="PS Scan Update", "Message Queue"=w253) -> ("dup Message Queue"=w252:refnum<queue>)  [unwired: 7 in, 1 out]
        n124 = local write "EIS Settings"(w238) -> ()
      }
      event "XYZ Velocity": Value Change {
        n125 = event-data() -> ()  [unwired: 1 in, 6 out]
        n126 = call-poly "Enqueue Message.vi"("Message Data"="XYZ Velocity", "Message"="Manual SET VEL", "Message Queue"=w257) -> ("dup Message Queue"=w256:refnum<queue>)  [unwired: 7 in, 1 out]
      }
      event "Start Range": Mouse Move {
        n127 = event-data() -> ("CtlRef"=w262:refnum<vi>, "Coords"=w261:T11)  [unwired: 1 in]
        n128 = invoke class="LstBox (strict)" method="Point To Row"(reference=w262, "Point"=w261) -> (reference out=w263:refnum<vi>, "InBounds"=w259:bool, "Row"=w260:i32)  [unwired: 5 in, 4 out]
        n129 = case shown="True" w259 {
          tunnel: w263 -> [_ w268]
          tunnel: w260 -> [_ w265]
          frame False {
          }
          frame True {
            n130 = property class="LstBox (strict)"(reference=w268, "Value"=w265) -> ()  [unwired: 1 in, 2 out]
            n131 = call "FGV Parameters.vi"("CMD"=PCT_FGV_CMD."SET", "input"=w265, "Key"="PS Start Range") -> ()  [unwired: 6 in, 3 out]
          }
        }
      }
      event "Current Range": Value Change {
        n132 = event-data() -> ("NewVal"=w269:i32[])  [unwired: 1 in]
        n133 = call "FGV Parameters.vi"("CMD"=PCT_FGV_CMD."SET", "input"=w269, "Key"="PS Range") -> ()  [unwired: 6 in, 3 out]
      }
    }
    n134 = call "Error Handler - Event Handling Loop.vi"("error in (no error)"=w29, "Message Queue"=w28) -> ("dup error in"=w30:errorcluster)  [unwired: 8 in, 1 out]
  }
  n135 = while {
    tunnel: w9 -> [w281]
    tunnel: w2 -> [w280]
    tunnel: w1 -> [w273]
    stop <- w284 stop-if-true
    n136 = Get Notifier Status(notifier=w273) -> (current notification=→"Actual Time":dbl)  [unwired: 1 in, 4 out]
    n137 = Unbundle By Name("PS Live Curve Result") -> ("Curve Values.Values"=→"PS XY Graph":cluster{"X Value":dbl, "Y Value":dbl}[])
    n138 = Wait on Notification(notifier=w280, timeout in ms (-1)=50) -> (notification=w277:cluster{"Timestamp  Stimulus   Value":dbl[][]}[], timed out?=w278:bool)  [unwired: 2 in, 2 out]
    n139 = case shown="True" "Timer Run" {
      tunnel: w281 -> [_ w293]
      frame False {
      }
      frame True {
        n140 = Get Notifier Status(notifier=w293) -> (current notification=w292:dbl[])  [unwired: 1 in, 4 out]
        n141 = Index Array(array=w292) -> (element=→"Test Time 3":dbl)  [unwired: 1 in]
      }
    }
    n142 = case shown="False" w278 {
      tunnel: w277 -> [w287 _]
      frame False {
        n143 = Index Array(array=w287) -> (element=w289:cluster{"Timestamp  Stimulus   Value":dbl[][]})  [unwired: 1 in]
        n144 = Unbundle By Name(w289) -> ("Timestamp  Stimulus   Value"=w290:dbl[][])
        n145 = Index Array(array=w290, index (col)=2 ("disabled index (col)")) -> (element=→"Waveform Chart 2":dbl[])  [unwired: 1 in]
      }
      frame True {
      }
    }
    n146 = call "FGV STOP.vi"("CMD"=PCT_FGV_CMD."GET") -> ("output"=w284:bool)  [unwired: 9 in, 1 out]
    n147 = Wait Until Next ms Multiple(millisecond multiple=u32 50) -> ()  [unwired: 1 out]
  }
  n148 = while "Data Display Loop" {
    tunnel: w14 -> [w308]
    tunnel: w11 -> [w303]
    tunnel: w8 -> [w301]
    tunnel: w6 -> [w302]
    tunnel: w5 -> [_]
    stop <- w315 stop-if-true
    # "Data Display Loop"
    n149 = Get Notifier Status(notifier=w303) -> ()  [unwired: 1 in, 5 out]
    n150 = Get Notifier Status(notifier=w302) -> ()  [unwired: 1 in, 5 out]
    n151 = Get Notifier Status(notifier=w301) -> (current notification=w296:cluster{"dX":dbl, "dY":dbl, "dZ":dbl, "dA":dbl})  [unwired: 1 in, 4 out]
    n152 = Wait Until Next ms Multiple(millisecond multiple=u32 1000) -> ()  [unwired: 1 out]
    n153 = Dequeue Element(queue=w308, timeout in ms (-1)=1000) -> (queue out=w306:refnum<queue>, element=w305:T13, timed out?=w304:bool)  [unwired: 1 in, 1 out]
    n154 = call "FGV GAGE Zero.vi"("CMD"=PCT_FGV_CMD."GET") -> ("output"=w299:dbl[])  [unwired: 9 in, 1 out]
    n155 = Unbundle By Name(w296) -> ("dX"=w297:dbl)
    n156 = call "UI Get time.vi"() -> ("Time"=→"Test Time 2":dbl, "Time Clusterr"=→"Timer":cluster{dbl, dbl, dbl})  [unwired: 10 in]
    n157 = Index Array(array=w299) -> (element=w298:dbl)  [unwired: 1 in]
    n158 = Subtract(x=w298, y=w297) -> (x-y=w295:dbl)
    n159 = Bundle By Name(cluster=w296, "dX"=w295) -> (→"Actual Position":cluster{"dX":dbl, "dY":dbl, "dZ":dbl, "dA":dbl})
    n160 = case shown="False" w304 {
      tunnel: w306 -> [_ _]
      tunnel: w305 -> [w318 _]
      frame False {
        n161 = for {
          tunnel: w318 -> [w325] mode=indexing
          tunnel: [w319] -> w317 mode=concatenating
          n162 = Unbundle By Name(w325) -> ("Curve Values.Values"=w324:cluster{"X Value":dbl, "Y Value":dbl}[])
          n163 = for {
            tunnel: w324 -> [w328] mode=indexing
            tunnel: [w327] -> w323 mode=indexing
            tunnel: [w326] -> w321 mode=indexing
            n164 = Unbundle By Name(w328) -> ("X Value"=w327:dbl, "Y Value"=w326:dbl)
          }
          n165 = call "Convert to Dynamic Data"("Array"=w323) -> ("Dynamic Data Type"=w322:dynamicdata)  [unwired: 3 in]
          n166 = call "Convert to Dynamic Data2"("Array"=w321) -> ("Dynamic Data Type"=w320:dynamicdata)  [unwired: 3 in]
          n167 = call "Build XY Graph"("Y Input"=w320, "X Input"=w322) -> ("XY Graph"=w319:cluster{"X":dbl[], "Y":dbl[]}[])  [unwired: 8 in, 1 out]
        }
        "PS Data" <- w317
      }
      frame True {
      }
    }
    n168 = call "FGV STOP.vi"("CMD"=PCT_FGV_CMD."GET") -> ("output"=w315:bool)  [unwired: 9 in, 1 out]
    n169 = Get Date/Time String(want seconds? (F)=TRUE) -> (date string=→"Date Display":string, time string=→"Time Display":string)  [unwired: 2 in]
  }
  n170 = call "Modules.vi"("VI in"=w16, "error in (no error)"=w21, "Stop Event"=w20) -> ("error out"=w15:errorcluster, "User Event out"=w19:refnum<user-event>)  [unwired: 7 in]
  n171 = Unregister For Events(event registration refnum=w25, error in=w26) -> (error out=w22:errorcluster)
  n172 = Merge Errors(w22, w15) -> (w23:errorcluster)
  n173 = call "RTS Shutdown.vi"("Stop Event"=w19, "error in"=w23) -> ("error out"=w24:errorcluster)  [unwired: 9 in]
  n174 = disable-structure shown="RUN_TIME_ENGINE==True" {
    disable-tunnel: w24 -> [_ _]
    frame condition #0 (active) {
    }
    frame condition #1 {
      # "Call Quit LabVIEW if running as a built application."
      n175 = Quit LabVIEW() -> ()  [unwired: 1 in]
    }
  }
  "DB" <- w10
  "PLC" <- w10
  "Motor Status" <- FALSE ("DMM GR Status")
  "String 9" <- "V 2.0.2" ("String 9")
